vi "End Arduino Comms.vi"(1 "Resource index":i32) -> (0 "Error":errorcluster)   [LabVIEW 2014]
uses:
  Arduino_comms_Global.vi
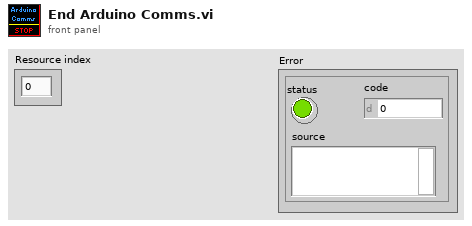
[diagram p1: front panel]
types:
  T1 = typedef "Arduino Config & resource typedef.ctl" = cluster{"VISA resource name":refnum<visa-resource-name>, "baud rate (bps)":u32, "timeout (ms)":u32, "data bits":u16, "parity":enum16{"None", "Odd", "Even", "Mark", "Space"}, "stop bits (10: 1 bit)":u16, "flow control":u16, "termination char (hex)":u8, "Enable Termination Char":bool, "byte count":u32, "Resource locked?":bool}
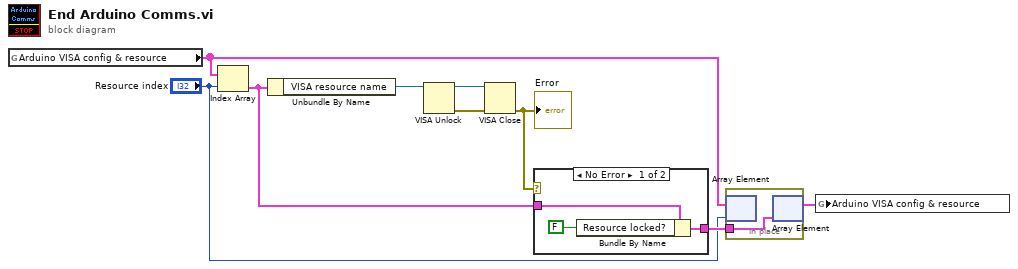
[diagram p0: block diagram]
diagram:
  n1 = global read "Arduino_comms_Global.vi" "Arduino VISA config & resource"() -> (w3:T1[])
  n2 = Index Array(array=w3, index="Resource index") -> (element=w5:T1)
  n3 = Unbundle By Name(w5) -> ("VISA resource name"=w7:refnum<visa-resource-name>)
  n4 = VISA Unlock(11:w7) -> (0:w9:errorcluster, 3:w8:refnum<visa-resource-name>)  [unwired: 1 in]
  n5 = VISA Close(VISA resource name=w8, error in (no error)=w9) -> (error out=w6:errorcluster)
  "Error" <- w6
  n6 = case shown="No Error" w6 {
    tunnel: [w10 w13] -> w4
    tunnel: w5 -> [w11 w13]
    frame No Error {
      n7 = Bundle By Name(cluster=w11, "Resource locked?"=FALSE ("Locked")) -> (w10:T1)
    }
    frame Error {
    }
  }
  n8 = in-place {
    in-place-border: w4 -> [w14]
    n9 = in-place-array #1(w3, "Resource index") -> ()  [unwired: 1 out]
    n10 = in-place-array #1(w14) -> (w2:T1[])  [unwired: 1 out]
  }
  n11 = global write "Arduino_comms_Global.vi" "Arduino VISA config & resource"(w2) -> ()
